vi "Kan Bağışı 2.vi"() -> ()   [LabVIEW 2017]
uses:
  <vilib>/Utility/file.llb/Read Delimited Spreadsheet (string).vi
panel:
  in  "Kan Grubu Seçiniz":string(combo)
  out "Baðýþçý Bilgileri":T1(array[cluster])
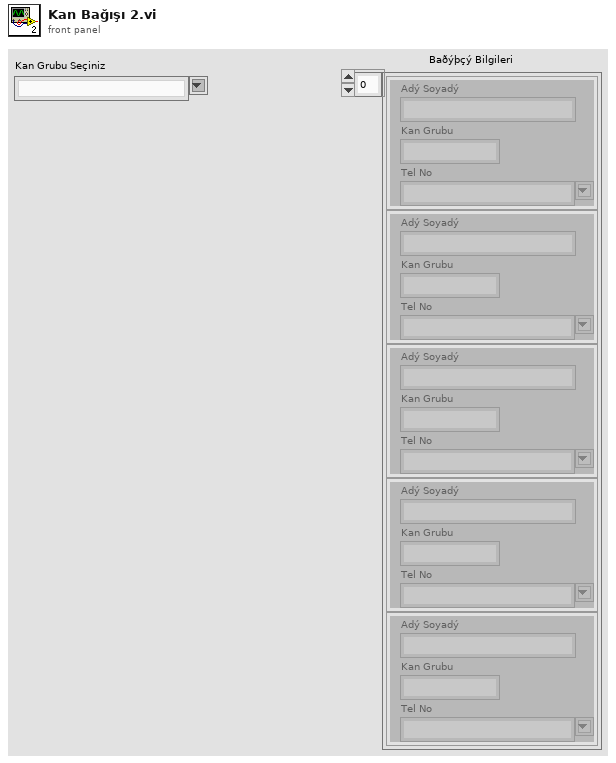
[diagram p1: front panel]
types:
  T1 = cluster{"Adý Soyadý":string, "Kan Grubu":string, "Tel No":string}[]
  T2 = cluster{"String":string, "String 2":string, "Combo Box":string}
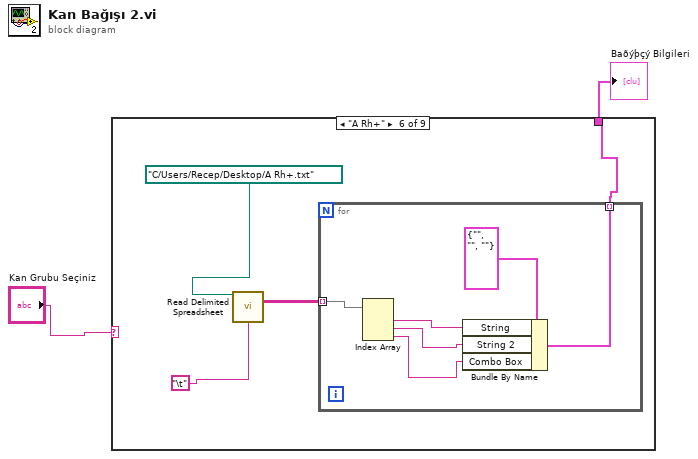
[diagram p0: block diagram]
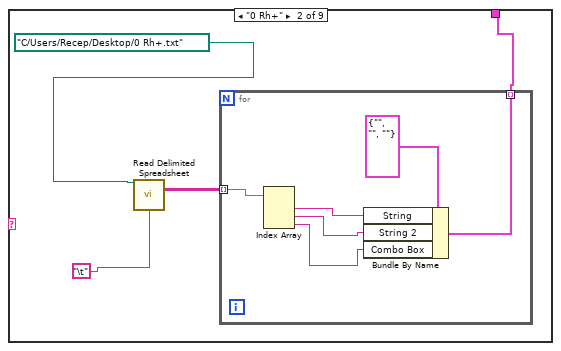
[diagram p3: hidden frame]
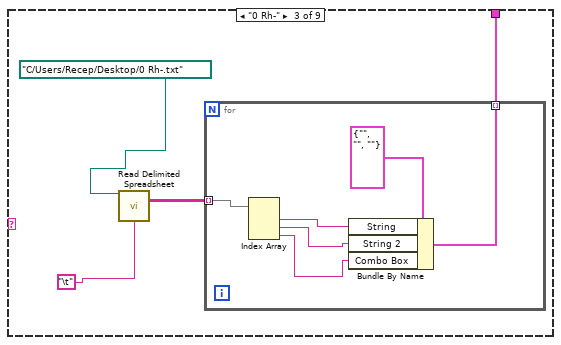
[diagram p4: hidden frame]
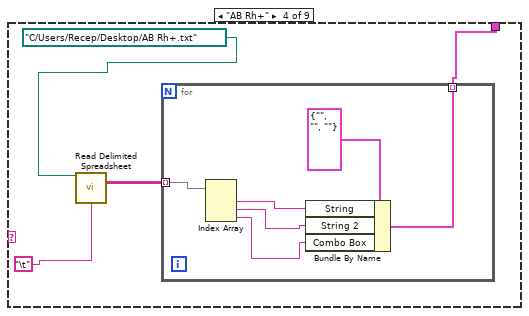
[diagram p5: hidden frame]
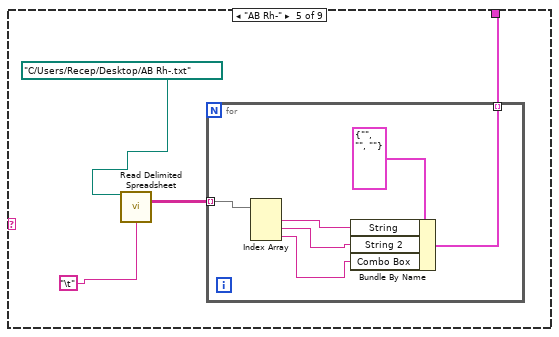
[diagram p6: hidden frame]
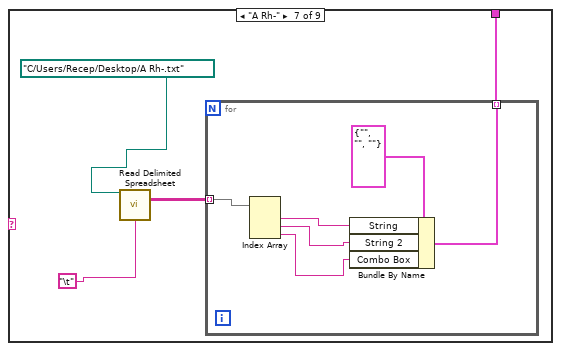
[diagram p7: hidden frame]
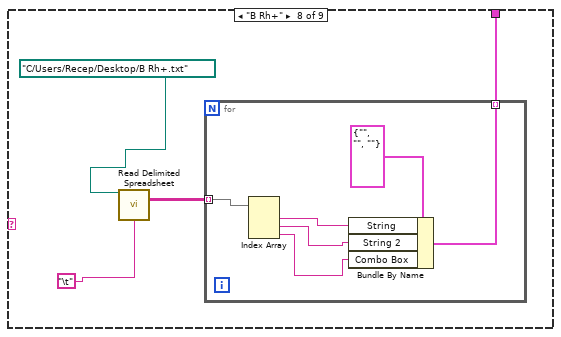
[diagram p8: hidden frame]
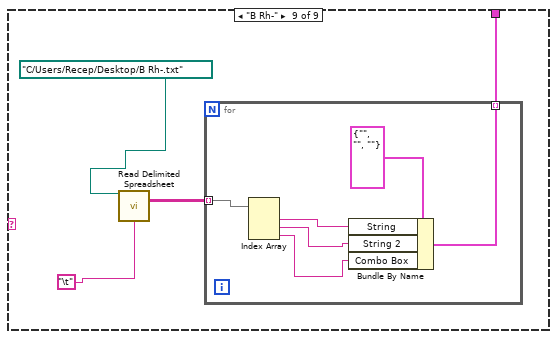
[diagram p9: hidden frame]
diagram:
  n1 = case shown="\"A Rh+\"" "Kan Grubu Seçiniz" {
    tunnel: [_ w4 w13 w24 w33 w44 w53 w64 w73] -> w2
    frame "False", Default {
    }
    frame "0 Rh+" {
      n2 = call-poly <vilib>:"Read Delimited Spreadsheet.vi"("file path (dialog if empty)"=path "C:/Users/Recep/Desktop/0 Rh+.txt" ("Path"), "delimiter (\\t)"="\t") -> ("all rows"=w5:string[][])  [unwired: 8 in, 5 out]
      n3 = for {
        tunnel: w5 -> [w12] mode=indexing
        tunnel: [w7] -> w4 mode=indexing
        n4 = Index Array(array=w12) -> (element #1=w11:string, element #2=w9:string, element #3=w8:string)  [unwired: 3 in]
        n5 = Bundle By Name(cluster=T2 {"String"="", "String 2"="", "Combo Box"=""} ("Cluster"), "String"=w11, "String 2"=w9, "Combo Box"=w8) -> (w7:T2)
      }
    }
    frame "0 Rh-" {
      n6 = call-poly <vilib>:"Read Delimited Spreadsheet.vi"("file path (dialog if empty)"=path "C:/Users/Recep/Desktop/0 Rh-.txt" ("Path"), "delimiter (\\t)"="\t") -> ("all rows"=w15:string[][])  [unwired: 8 in, 5 out]
      n7 = for {
        tunnel: w15 -> [w22] mode=indexing
        tunnel: [w17] -> w13 mode=indexing
        n8 = Index Array(array=w22) -> (element #1=w21:string, element #2=w19:string, element #3=w18:string)  [unwired: 3 in]
        n9 = Bundle By Name(cluster=T2 {"String"="", "String 2"="", "Combo Box"=""} ("Cluster"), "String"=w21, "String 2"=w19, "Combo Box"=w18) -> (w17:T2)
      }
    }
    frame "AB Rh+" {
      n10 = call-poly <vilib>:"Read Delimited Spreadsheet.vi"("file path (dialog if empty)"=path "C:/Users/Recep/Desktop/AB Rh+.txt" ("Path"), "delimiter (\\t)"="\t") -> ("all rows"=w25:string[][])  [unwired: 8 in, 5 out]
      n11 = for {
        tunnel: w25 -> [w32] mode=indexing
        tunnel: [w27] -> w24 mode=indexing
        n12 = Index Array(array=w32) -> (element #1=w31:string, element #2=w29:string, element #3=w28:string)  [unwired: 3 in]
        n13 = Bundle By Name(cluster=T2 {"String"="", "String 2"="", "Combo Box"=""} ("Cluster"), "String"=w31, "String 2"=w29, "Combo Box"=w28) -> (w27:T2)
      }
    }
    frame "AB Rh-" {
      n14 = call-poly <vilib>:"Read Delimited Spreadsheet.vi"("file path (dialog if empty)"=path "C:/Users/Recep/Desktop/AB Rh-.txt" ("Path"), "delimiter (\\t)"="\t") -> ("all rows"=w35:string[][])  [unwired: 8 in, 5 out]
      n15 = for {
        tunnel: w35 -> [w42] mode=indexing
        tunnel: [w37] -> w33 mode=indexing
        n16 = Index Array(array=w42) -> (element #1=w41:string, element #2=w39:string, element #3=w38:string)  [unwired: 3 in]
        n17 = Bundle By Name(cluster=T2 {"String"="", "String 2"="", "Combo Box"=""} ("Cluster"), "String"=w41, "String 2"=w39, "Combo Box"=w38) -> (w37:T2)
      }
    }
    frame "A Rh+" {
      n18 = call-poly <vilib>:"Read Delimited Spreadsheet.vi"("file path (dialog if empty)"=path "C:/Users/Recep/Desktop/A Rh+.txt" ("Path"), "delimiter (\\t)"="\t") -> ("all rows"=w45:string[][])  [unwired: 8 in, 5 out]
      n19 = for {
        tunnel: w45 -> [w52] mode=indexing
        tunnel: [w47] -> w44 mode=indexing
        n20 = Index Array(array=w52) -> (element #1=w51:string, element #2=w49:string, element #3=w48:string)  [unwired: 3 in]
        n21 = Bundle By Name(cluster=T2 {"String"="", "String 2"="", "Combo Box"=""} ("Cluster"), "String"=w51, "String 2"=w49, "Combo Box"=w48) -> (w47:T2)
      }
    }
    frame "A Rh-" {
      n22 = call-poly <vilib>:"Read Delimited Spreadsheet.vi"("file path (dialog if empty)"=path "C:/Users/Recep/Desktop/A Rh-.txt" ("Path"), "delimiter (\\t)"="\t") -> ("all rows"=w55:string[][])  [unwired: 8 in, 5 out]
      n23 = for {
        tunnel: w55 -> [w62] mode=indexing
        tunnel: [w57] -> w53 mode=indexing
        n24 = Index Array(array=w62) -> (element #1=w61:string, element #2=w59:string, element #3=w58:string)  [unwired: 3 in]
        n25 = Bundle By Name(cluster=T2 {"String"="", "String 2"="", "Combo Box"=""} ("Cluster"), "String"=w61, "String 2"=w59, "Combo Box"=w58) -> (w57:T2)
      }
    }
    frame "B Rh+" {
      n26 = call-poly <vilib>:"Read Delimited Spreadsheet.vi"("file path (dialog if empty)"=path "C:/Users/Recep/Desktop/B Rh+.txt" ("Path"), "delimiter (\\t)"="\t") -> ("all rows"=w65:string[][])  [unwired: 8 in, 5 out]
      n27 = for {
        tunnel: w65 -> [w72] mode=indexing
        tunnel: [w67] -> w64 mode=indexing
        n28 = Index Array(array=w72) -> (element #1=w71:string, element #2=w69:string, element #3=w68:string)  [unwired: 3 in]
        n29 = Bundle By Name(cluster=T2 {"String"="", "String 2"="", "Combo Box"=""} ("Cluster"), "String"=w71, "String 2"=w69, "Combo Box"=w68) -> (w67:T2)
      }
    }
    frame "B Rh-" {
      n30 = call-poly <vilib>:"Read Delimited Spreadsheet.vi"("file path (dialog if empty)"=path "C:/Users/Recep/Desktop/B Rh-.txt" ("Path"), "delimiter (\\t)"="\t") -> ("all rows"=w75:string[][])  [unwired: 8 in, 5 out]
      n31 = for {
        tunnel: w75 -> [w82] mode=indexing
        tunnel: [w77] -> w73 mode=indexing
        n32 = Index Array(array=w82) -> (element #1=w81:string, element #2=w79:string, element #3=w78:string)  [unwired: 3 in]
        n33 = Bundle By Name(cluster=T2 {"String"="", "String 2"="", "Combo Box"=""} ("Cluster"), "String"=w81, "String 2"=w79, "Combo Box"=w78) -> (w77:T2)
      }
    }
  }
  "Baðýþçý Bilgileri" <- w2
